vi "Write Next Row.vi"(8 "error in (no error)":errorcluster, 10 "Next Row":i32, 11 "PQ Result  in":refnum<class "PQ Result.lvclass">) -> (0 "error out":errorcluster, 3 "PQ Result  out":refnum<class "PQ Result.lvclass">)   [LabVIEW 2016, in "PQ Result.lvclass"]
uses:
  PQ Result.lvclass
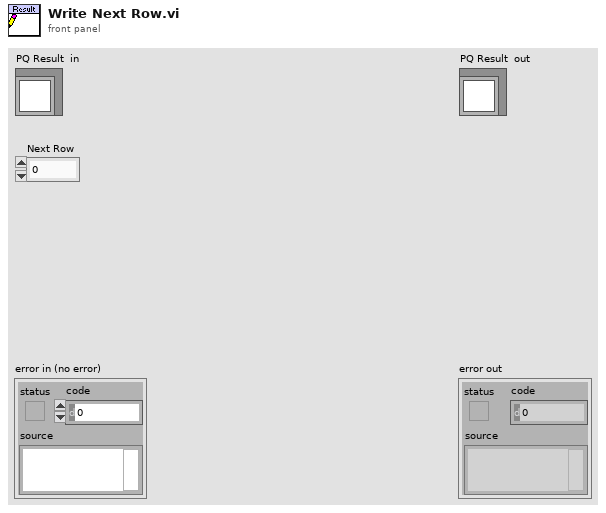
[diagram p1: front panel]
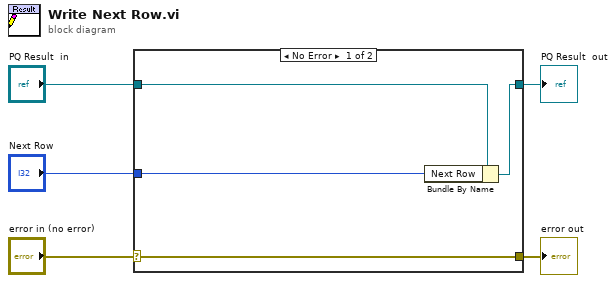
[diagram p0: block diagram]
diagram:
  n1 = case shown="No Error" "error in (no error)" {
    selector: "error in (no error)" -> [w9 w10]
    tunnel: [w9 w10] -> w4
    tunnel: [w7 w11] -> w2
    tunnel: "PQ Result  in" -> [w8 w11]
    tunnel: "Next Row" -> [w6 _]
    frame No Error {
      n2 = Bundle By Name(cluster=w8, "Next Row"=w6) -> (w7:refnum<class "PQ Result.lvclass">)
    }
    frame Error {
    }
  }
  "error out" <- w4
  "PQ Result  out" <- w2
